vi "Basic Function Generator.vi"(0 "frequency":dbl=10.0 format="%0.2p", 1 "signal type":T1(ring), 3 "reset signal":bool, 4 "offset":dbl format="%0.2p", 5 "amplitude":dbl=1.0 format="%0.2p", 9 "phase":dbl format="%.2p", 11 "error in (no error)":errorcluster, 12 "sampling info":cluster{"Fs":dbl, "#s":dbl}={"Fs"=1000.0, "#s"=1000.0} {"Fs" format="%.2p"}, 13 "square wave duty cycle (%)":dbl=50.0 format="%0.2f") -> (6 "signal out":waveform(dbl), 8 "DBL Out":dbl[](array[numeric]), 10 "phase out":dbl format="%.2p", 15 "error out":errorcluster)   [LabVIEW 2010]
doc: "Creates an output waveform based on <B>signal type</B>."
uses:
  <vilib>/measure/maUtilsandCtls.llb/ma_Updatet0 timestamp.vi
  <vilib>/measure/NI_MABase.lvlib
  <vilib>/Analysis/NI_AALBase.lvlib
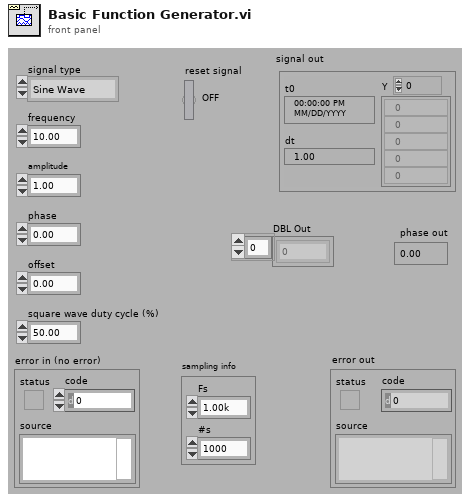
[diagram p1: front panel]
types:
  T1 = enum16{"Sine Wave", "Triangle Wave", "Square Wave", "Sawtooth Wave"}
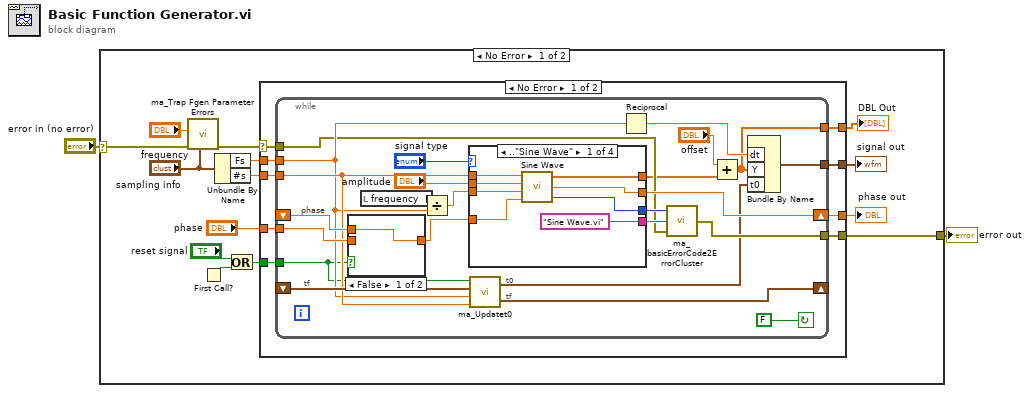
[diagram p0: block diagram]
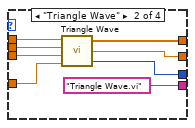
[diagram p2: hidden frame]
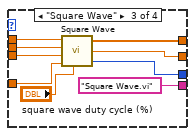
[diagram p3: hidden frame]
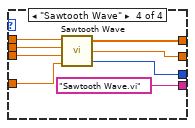
[diagram p4: hidden frame]
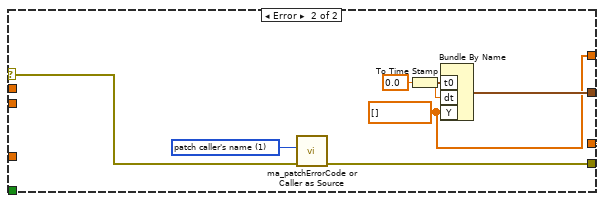
[diagram p6: hidden frame]
diagram:
  n1 = case shown="No Error" "error in (no error)" {
    selector: "error in (no error)" -> [w4 w93]
    tunnel: [w15 w93] -> w2
    frame No Error {
      n2 = call <vilib>:"ma_Trap Fgen Parameter Errors.vi"("Sampling info"="sampling info", "error in (no error)"=w4, "frequency"="frequency") -> ("error out"=w14:errorcluster)  [unwired: 8 in]
      n3 = First Call?() -> (First Call?: T/F=w8:bool)
      n4 = Unbundle By Name("sampling info") -> ("Fs"=w10:dbl, "#s"=w9:dbl)
      n5 = Or(x="reset signal", y=w8) -> (x .or. y?=w6:bool)
      n6 = case shown="No Error" w14 {
        selector: w14 -> [w18 w88]
        tunnel: [w25 w92] -> w16
        tunnel: [w24 w87] -> w15
        tunnel: "phase" -> [w23 _]
        tunnel: w10 -> [w22 _]
        tunnel: w9 -> [w21 _]
        tunnel: w6 -> [w20 _]
        tunnel: [w19 w90] -> w5
        tunnel: [w17 w85] -> w3
        frame No Error {
          n7 = while {
            tunnel: w18 -> [w30]
            tunnel: [w33] -> w19
            tunnel: w20 -> [w34]
            tunnel: w21 -> [w36]
            tunnel: w22 -> [w35]
            tunnel: w23 -> [w46]
            tunnel: [w29] -> w24
            shift-left: _ -> [w49]
            shift-right: [w38] -> w25
            shift-left: _ -> [w47]
            shift-right: [w48] -> _
            tunnel: [w26] -> w17
            stop <- FALSE continue-if-true
            # "tf"
            # "t0"
            # "phase"
            # "tf"
            n8 = case shown="False" w34 {
              tunnel: w49 -> [w83 _]
              tunnel: [w83 w84] -> w41
              tunnel: w46 -> [_ w84]
              frame False {
              }
              frame True {
              }
            }
            n9 = local read "frequency"() -> (w40:dbl)
            n10 = Divide(x=w40, y=w35) -> (x/y=w43:dbl)
            n11 = case shown="..\"Sine Wave\"" "signal type" {
              tunnel: w43 -> [w57 w65 w74 w82]
              tunnel: "amplitude" -> [w56 w64 w73 w81]
              tunnel: w36 -> [w55 w63 w72 w80]
              tunnel: w41 -> [w54 w62 w71 w79]
              tunnel: [w53 w61 w70 w78] -> w38
              tunnel: [w52 w60 w69 w77] -> w27
              tunnel: ["Sine Wave.vi" ("subVI Name") "Triangle Wave.vi" ("subVI Name") "Square Wave.vi" ("subVI Name") "Sawtooth Wave.vi" ("subVI Name")] -> w32
              tunnel: [w51 w59 w67 w75] -> w31
              frame .."Sine Wave" {
                n12 = call <vilib>:"Sine Wave.vi"("samples"=w55, "amplitude"=w56, "frequency"=w57, "phase in"=w54) -> ("sine wave"=w52:dbl[], "phase out"=w53:dbl, "error"=w51:i32)  [unwired: 1 in]
              }
              frame "Triangle Wave" {
                n13 = call <vilib>:"Triangle Wave.vi"("samples"=w63, "amplitude"=w64, "frequency"=w65, "phase in"=w62) -> ("triangle wave"=w60:dbl[], "phase out"=w61:dbl, "error"=w59:i32)  [unwired: 1 in]
              }
              frame "Square Wave" {
                n14 = call <vilib>:"Square Wave.vi"("samples"=w72, "amplitude"=w73, "frequency"=w74, "duty cycle (%)"="square wave duty cycle (%)", "phase in"=w71) -> ("square wave"=w69:dbl[], "phase out"=w70:dbl, "error"=w67:i32)  [unwired: 1 in]
              }
              frame "Sawtooth Wave" {
                n15 = call <vilib>:"Sawtooth Wave.vi"("samples"=w80, "amplitude"=w81, "frequency"=w82, "phase in"=w79) -> ("sawtooth wave"=w77:dbl[], "phase out"=w78:dbl, "error"=w75:i32)  [unwired: 1 in]
              }
            }
            n16 = call-poly <vilib>:"ma_Updatet0.vi"("samples"=w36, "sampling rate (S/s)"=w35, "tf previous"=w47, "Reset Generation"=w34) -> ("tf new"=w48:timestamp, "t0"=w28:timestamp)
            n17 = Reciprocal(x=w35) -> (1/x=w44:dbl)
            n18 = call <vilib>:"ma_basicErrorCode2ErrorCluster.vi"("error in (no error)"=w30, "subVI name"=w32, "Error Code"=w31) -> ("error out"=w29:errorcluster)
            n19 = Add(x="offset", y=w27) -> (x+y=w26:dbl[])
            n20 = Bundle By Name("dt"=w44, "Y"=w26, "t0"=w28) -> (w33:waveform(dbl))  [unwired: 1 in]
          }
        }
        frame Error {
          w86 = u16 1 items=["patch error code", "patch caller's name"] ("operation")
          w85 = dbl[] [] ("Y")
          w91 = 0.0 ("t0")
          w92 = 0.0  # phase out
          n21 = call <vilib>:"ma_patchErrorCode or Caller as Source.vi"("error in (no error)"=w88, "operation"=w86) -> ("error out"=w87:errorcluster)  [unwired: 9 in]
          n22 = To Time Stamp(1:w91) -> (0:w89:timestamp)
          n23 = Bundle By Name("t0"=w89, "dt"=w91, "Y"=w85) -> (w90:waveform(dbl))  [unwired: 1 in]
        }
      }
      "phase out" <- w16
      "signal out" <- w5
      "DBL Out" <- w3
    }
    frame Error {
    }
  }
  "error out" <- w2
